vi "Agilent U2000 Series Acquire Reference Trace.vi"() -> ()   [LabVIEW 2018]
doc: "This example shows how to acquire the reference trace data using the VIs on this driver.\n\nNote:\nThis example is applicable for U2021/2XA only."
uses:
  Public/Data/Read CCDF (Reference Trace).vi
  Agilent U2000 Series.lvlib
panel:
  out "Reference Trace Data":dbl[](array[numeric])
  out "Peak-to-average Data":dbl
  out "Average Power Data":dbl
  out "Max X-axis Value (dB)":i32
  out "Peak Power Data":dbl
  in  "VISA resource name":refnum<visa-resource-name>
  # "(c) 2011-2015 National Instruments.  ALL RIGHTS RESERVED."
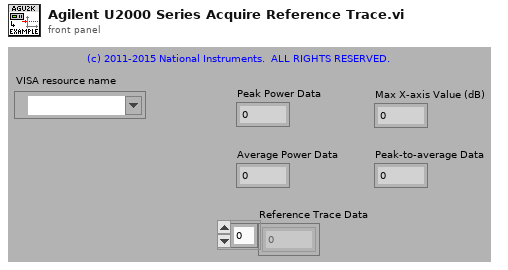
[diagram p1: front panel]
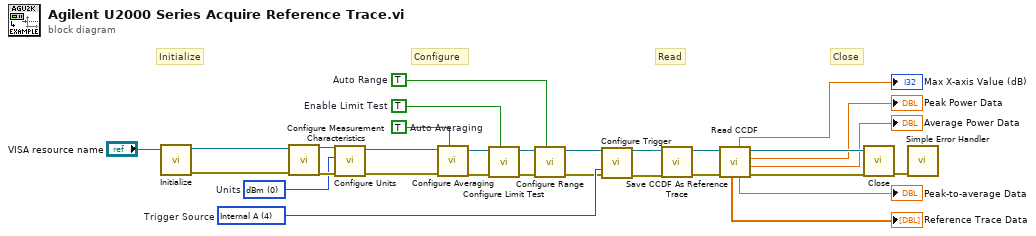
[diagram p0: block diagram]
diagram:
  w23 = 4 items=["Bus", "External", "Hold", "Immediate", "Internal A"]  # Trigger Source
  w16 = TRUE  # Enable Limit Test
  w24 = u16 0 items=["dBm", "W"]  # Units
  w17 = TRUE  # Auto Averaging
  w15 = TRUE  # Auto Range
  # "Close"
  # "Read"
  # "Configure"
  # "Initialize"
  n1 = call "Initialize.vi"("VISA resource name"="VISA resource name") -> ("error out"=w27:errorcluster, "VISA resource name out"=w28:refnum<visa-resource-name>)  [unwired: 3 in, 6 out]
  n2 = call "Configure Measurement Characteristics.vi"("VISA resource name"=w28, "error in (no error)"=w27) -> ("VISA resource name out"=w26:refnum<visa-resource-name>, "error out"=w25:errorcluster)  [unwired: 12 in]
  n3 = call "Configure Units.vi"("error in (no error)"=w25, "Units (0: dBm)"=w24, "VISA resource name"=w26) -> ("error out"=w20:errorcluster, "VISA resource name out"=w21:refnum<visa-resource-name>)  [unwired: 1 in, 6 out]
  n4 = call "Configure Averaging.vi"("Enable Averaging (T: Enable)"=w17, "error in (no error)"=w20, "VISA resource name"=w21) -> ("error out"=w18:errorcluster, "VISA resource name out"=w19:refnum<visa-resource-name>)  [unwired: 7 in]
  n5 = call "Configure Limit Test.vi"("Limit Test (T: Enable)"=w16, "error in (no error)"=w18, "VISA resource name"=w19) -> ("error out"=w13:errorcluster, "VISA resource name out"=w14:refnum<visa-resource-name>)  [unwired: 2 in, 5 out]
  n6 = call "Configure Range.vi"("Auto Range (T: Enable)"=w15, "error in (no error)"=w13, "VISA resource name"=w14) -> ("error out"=w12:errorcluster, "VISA resource name out"=w22:refnum<visa-resource-name>)  [unwired: 7 in]
  n7 = call "Configure Trigger.vi"("VISA resource name"=w22, "Trigger Source (3: Immediate)"=w23, "error in (no error)"=w12) -> ("VISA resource name out"=w10:refnum<visa-resource-name>, "error out"=w11:errorcluster)  [unwired: 5 in, 6 out]
  n8 = call "Save CCDF As Reference Trace.vi"("error in (no error)"=w11, "VISA resource name"=w10) -> ("error out"=w9:errorcluster, "VISA resource name out"=w8:refnum<visa-resource-name>)  [unwired: 8 out]
  n9 = call-poly "Read CCDF.vi"("error in (no error)"=w9, "VISA resource name"=w8) -> ("error out"=w6:errorcluster, "Average Power Data"=→"Average Power Data":dbl, "Max X-axis Value (dB)"=→"Peak Power Data":dbl, "VISA resource name out"=w7:refnum<visa-resource-name>, "Peak-to-average Data"=→"Peak-to-average Data":dbl, "Peak Power Data"=→"Max X-axis Value (dB)":dbl, "Reference Trace Data"=→"Reference Trace Data":dbl[])  [unwired: 3 in]
  n10 = call "Close.vi"("error in (no error)"=w6, "VISA resource name"=w7) -> ("error out"=w29:errorcluster)  [unwired: 9 out]
  n11 = call <vilib>:"Simple Error Handler.vi"("error in (no error)"=w29) -> ()  [unwired: 1 in, 8 out]
